vi "getCategoryByName.vi"(8 "error in (no error)":errorcluster, 10 "Name":string, 11 "Account History in":refnum<class "Account History.lvclass">) -> (0 "error out":errorcluster, 2 "Category.lvclass":refnum<class "Category.lvclass">, 3 "Account History out":refnum<class "Account History.lvclass">)   [LabVIEW 2018, in "Account History.lvclass"]
uses:
  Account History.lvclass
  Category/Category.lvclass
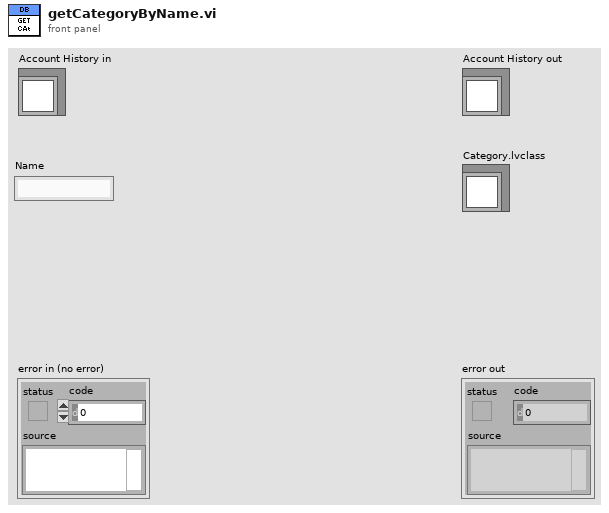
[diagram p1: front panel]
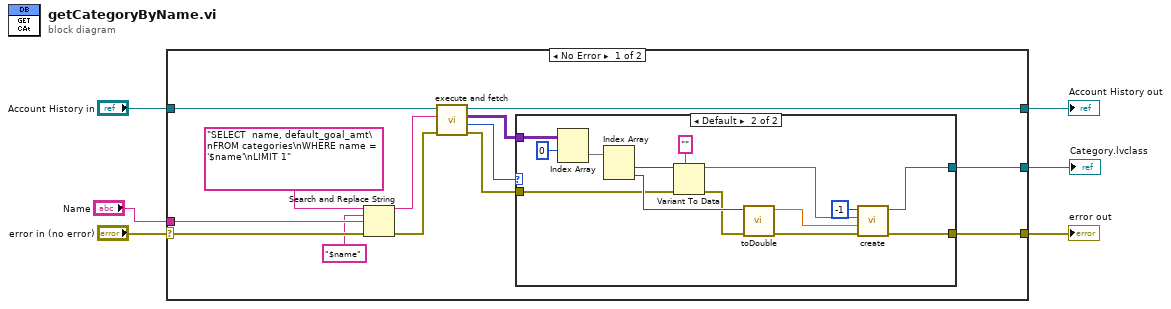
[diagram p0: block diagram]
diagram:
  n1 = case shown="No Error" "error in (no error)" {
    selector: "error in (no error)" -> [w16 w36]
    tunnel: [w10 w36] -> w5
    tunnel: [w18 w35] -> w3
    tunnel: "Account History in" -> [w19 w35]
    tunnel: "Name" -> [w15 _]
    tunnel: [w11 _] -> w1
    frame No Error {
      n2 = Search and Replace String(input string="SELECT  name, default_goal_amt\nFROM categories\nWHERE name = '$name'\nLIMIT 1", search string="$name", replace string=w15, error in=w16) -> (result string=w13:string, error out=w12:errorcluster)  [unwired: 4 in, 2 out]
      n3 = call "execute and fetch.vi"("error in (no error)"=w12, "SQL query"=w13, "Database in"=w19) -> ("error out"=w8:errorcluster, "Num records"=w7:i32, "recordset data"=w9:variant[][], "Database out"=w18:refnum<class "Account History.lvclass">)  [unwired: 5 in]
      n4 = case shown="Default" w7 {
        tunnel: [_ w34] -> w11
        tunnel: [w20 w33] -> w10
        tunnel: w9 -> [_ w32]
        tunnel: w8 -> [w20 w24]
        frame 0 {
        }
        frame Default {
          n5 = Index Array(array=w32, index (row)=0) -> (element=w30:variant[])  [unwired: 1 in]
          n6 = Index Array(array=w30) -> (element #1=w25:variant, element #2=w29:variant)  [unwired: 2 in]
          n7 = Variant To Data(error in=w24, type="", Variant=w25) -> (data=w21:string, error out=w23:errorcluster)
          n8 = call "toDouble.vi"("error in (no error)"=w23, "Value"=w29) -> ("error out"=w28:errorcluster, "type"=w27:dbl)  [unwired: 8 in]
          n9 = call "create.vi"("error in (no error)"=w28, "Default Goal Amount"=w27, "Name"=w21, "id"=-1) -> ("error out"=w33:errorcluster, "Category out"=w34:refnum<class "Category.lvclass">)  [unwired: 6 in]
        }
      }
    }
    frame Error {
    }
  }
  "error out" <- w5
  "Account History out" <- w3
  "Category.lvclass" <- w1
